vi "Percentiles.vi"   [LabVIEW 2020, in "NI_Gmath.lvlib"]
doc: "Computes a value that is greater than <B>p</B> percent of the data values in <B>x array</B>. Wire data to the <B>p</B> input to determine the polymorphic instance to use or manually select the instance."
uses:
  <vilib>/gmath/NI_Gmath.lvlib
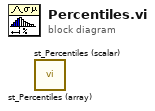
[diagram p0: block diagram]
diagram:
  n1 = call <vilib>:"st_Percentiles (array).vi"() -> ()  [unwired: 10 in, 2 out]
  n2 = call <vilib>:"st_Percentiles (scalar).vi"() -> ()  [unwired: 10 in, 2 out]
